vi "Replace and Reduce Array.vi"(6 "dimension size":i32=50, 7 "initialized 2D in":dbl[][](array[numeric]), 8 "error in":errorcluster, 9 "rows to display":i32, 10 "tc":u32, 11 "1D array":dbl[](array[numeric])) -> (0 "error out":errorcluster, 2 "start index":u32, 3 "reduced 2D":dbl[][](array[numeric]), 5 "initialized 2D out":dbl[][](array[numeric]))   [LabVIEW 2019, in "Zen Analytics.lvlib" / "Zen Analytics.lvclass"]
uses:
  Zen Analytics.lvclass
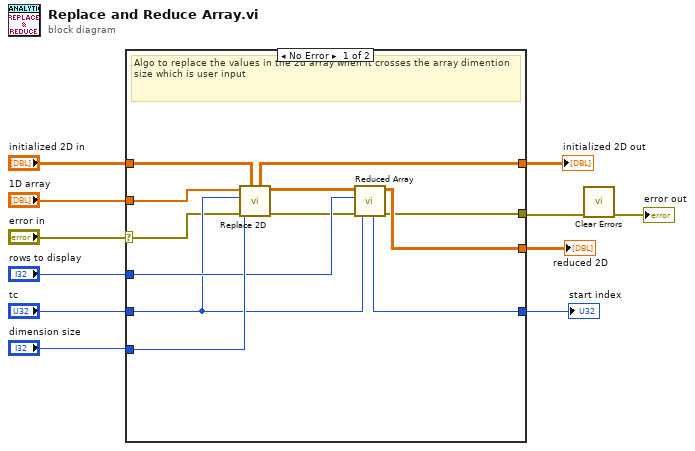
[diagram p0: block diagram]
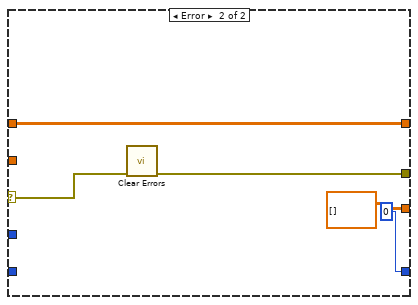
[diagram p2: hidden frame]
diagram:
  n1 = case shown="No Error" "error in" {
    selector: "error in" -> [w14 w27]
    tunnel: "dimension size" -> [w22 _]
    tunnel: "1D array" -> [w21 _]
    tunnel: "initialized 2D in" -> [w20 w26]
    tunnel: [w19 w26] -> w8
    tunnel: "rows to display" -> [w18 _]
    tunnel: "tc" -> [w17 _]
    tunnel: [w16 dbl[][] [] ("reduced array out")] -> w5
    tunnel: [w15 w23] -> w2
    tunnel: [w13 0 ("start index")] -> w3
    frame No Error {
      # "Algo to replace the values in the 2d array when it crosses the array dimention size which is user input"
      n2 = call "Replace 2D.vi"("initialized 2D in"=w20, "error in"=w14, "dimension size"=w22, "tc"=w17, "1D array"=w21) -> ("error out"=w12:errorcluster, "initialized 2D out"=w19:dbl[][])  [unwired: 5 in]
      n3 = call "Reduced Array.vi"("error in (no error)"=w12, "terminal count"=w17, "RTD"=w18, "initialized array in"=w19) -> ("error out"=w15:errorcluster, "start index"=w13:u32, "reduced array out"=w16:dbl[][])  [unwired: 5 in]
    }
    frame Error {
      n4 = call <vilib>:"Clear Errors.vi"("error in (no error)"=w27) -> ("error out"=w23:errorcluster)  [unwired: 5 in, 1 out]
    }
  }
  "initialized 2D out" <- w8
  "reduced 2D" <- w5
  "start index" <- w3
  n5 = call <vilib>:"Clear Errors.vi"("error in (no error)"=w2) -> ("error out"=→"error out":errorcluster)  [unwired: 5 in, 1 out]
